vi "Make Timestamped Segment.vi"(0 "TreeNode in":refnum<class "TreeNode.lvclass">, 5 "Segment data":refnum<class "Data.lvclass">, 7 "Timestamps":refnum<class "Int64Array.lvclass">, 9 "Array":i64[](array[numeric]), 11 "error in (no error)":errorcluster) -> (4 "TreeNode out":refnum<class "TreeNode.lvclass">, 15 "error out":errorcluster)   [LabVIEW 2015, in "MDSplus.lvlib" / "TreeNode.lvclass"]
doc: "Write a single row of timestamped data."
uses:
  <vilib>/MDSplus/Classes/Data_Class/TreeNode_Class/TreeNode.lvclass
  <vilib>/MDSplus/Classes/Data_Class/Data.lvclass
  <vilib>/MDSplus/Classes/Data_Class/Array_Class/Int64Array_Class/Int64Array.lvclass
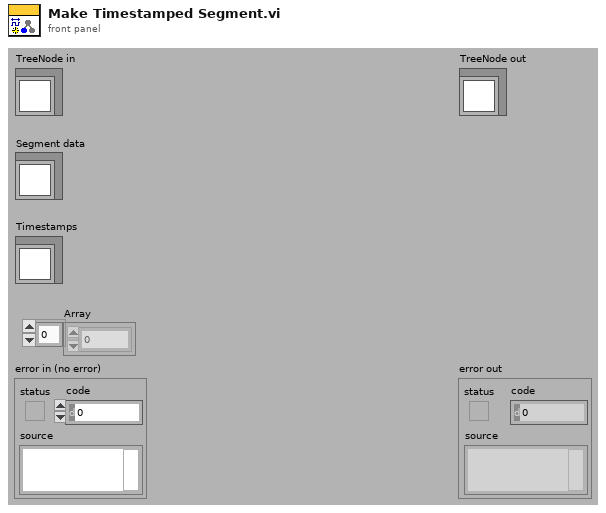
[diagram p1: front panel]
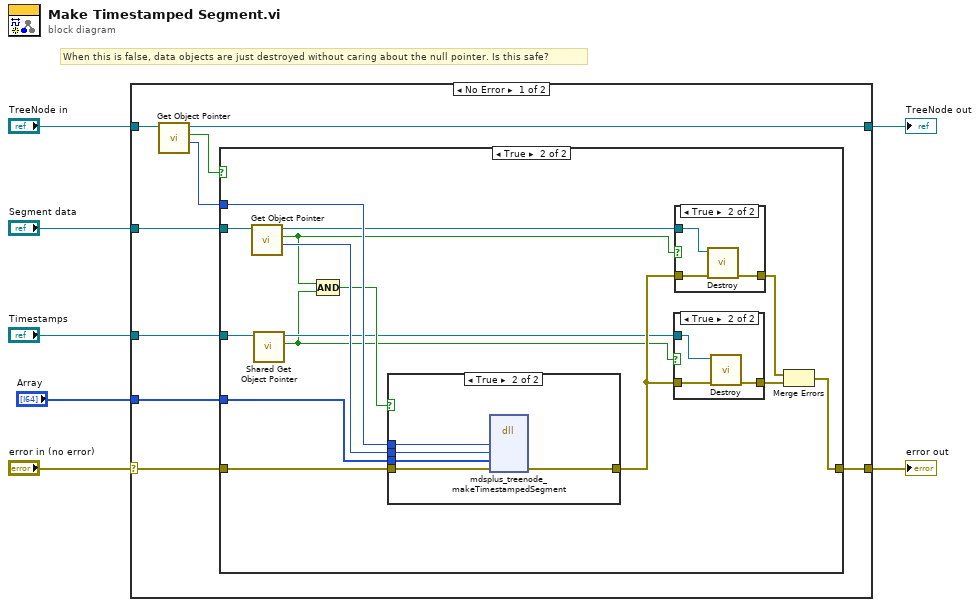
[diagram p0: block diagram]
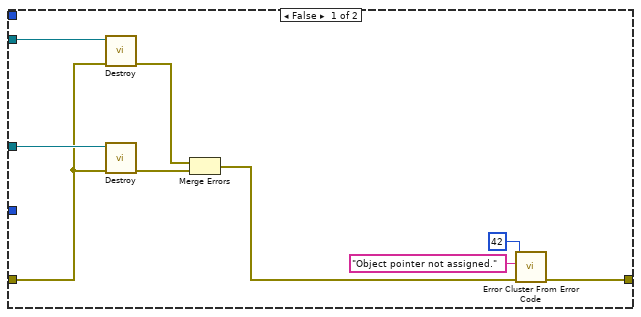
[diagram p2: hidden frame]
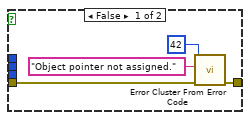
[diagram p5: hidden frame]
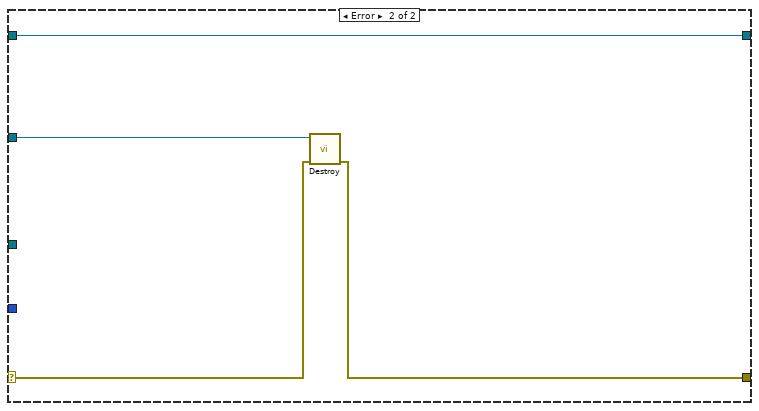
[diagram p6: hidden frame]
diagram:
  # "When this is false, data objects are just destroyed without caring about the null pointer. Is this safe?"
  n1 = case shown="No Error" "error in (no error)" {
    selector: "error in (no error)" -> [w12 w59]
    tunnel: [w11 w58] -> w6
    tunnel: [w10 w61] -> w4
    tunnel: "TreeNode in" -> [w16 w61]
    tunnel: "Segment data" -> [w15 w60]
    tunnel: "Timestamps" -> [w9 _]
    tunnel: "Array" -> [w8 _]
    frame No Error {
      n2 = call-dynamic "Get Object Pointer.vi"("Data in"=w16) -> ("Object Pointer"=w13:i64, "Assigned object pointer?"=w14:bool, "Data out"=w10:refnum<class "TreeNode.lvclass">)  [unwired: 8 in]
      n3 = case shown="True" w14 {
        tunnel: w15 -> [w22 w40]
        tunnel: w13 -> [_ w38]
        tunnel: w12 -> [w20 w37]
        tunnel: [w23 w27] -> w11
        tunnel: w9 -> [w21 w36]
        tunnel: w8 -> [_ w26]
        frame False {
          n4 = call-dynamic "Destroy.vi"("error in (no error)"=w20, "Data in"=w22) -> ("error out"=w19:errorcluster)  [unwired: 9 in]
          n5 = call-dynamic "Destroy.vi"("error in (no error)"=w20, "Int64Array in"=w21) -> ("error out"=w18:errorcluster)  [unwired: 9 in]
          n6 = Merge Errors(w19, w18) -> (w17:errorcluster)
          n7 = call <vilib>:"Error Cluster From Error Code.vi"("error in (no error)"=w17, "error message (\"\")"="Object pointer not assigned." ("error message (\"\")"), "error code (0)"=42) -> ("error out"=w23:errorcluster)  [unwired: 6 in]
        }
        frame True {
          n8 = call-dynamic "Get Object Pointer.vi"("Data in"=w40) -> ("Object Pointer"=w39:i64, "Assigned object pointer?"=w31:bool, "Data out"=w33:refnum<class "Data.lvclass">)  [unwired: 8 in]
          n9 = call <vilib>:"Shared Get Object Pointer.vi"("Data in"=w36) -> ("Assigned object pointer?"=w30:bool, "Data out"=w32:refnum<class "Int64Array.lvclass">)  [unwired: 8 in, 1 out]
          n10 = Compound Arithmetic op=AND(w31, w30) -> (w35:bool)
          n11 = case shown="True" w35 {
            tunnel: w39 -> [_ w53]
            tunnel: w38 -> [_ w56]
            tunnel: w37 -> [w49 w57]
            tunnel: [w50 w54] -> w34
            tunnel: w26 -> [_ w55]
            frame False {
              n12 = call <vilib>:"Error Cluster From Error Code.vi"("error in (no error)"=w49, "error message (\"\")"="Object pointer not assigned." ("error message (\"\")"), "error code (0)"=42) -> ("error out"=w50:errorcluster)  [unwired: 6 in]
            }
            frame True {
              n13 = dll-call lib="MDSobjectsLVShr" fn="mdsplus_treenode_makeTimestampedSegment"("lvTreeNodePtr"=w56, "lvArrayPtrIn"=w53, "lvLngArrHdlIn"=w55, "error"=w57) -> ("error"=w54:errorcluster)  [unwired: 7 in, 2 out]
            }
          }
          n14 = case shown="True" w30 {
            tunnel: w34 -> [w45 w48]
            tunnel: w32 -> [_ w46]
            tunnel: [w45 w47] -> w28
            frame False {
            }
            frame True {
              n15 = call-dynamic "Destroy.vi"("error in (no error)"=w48, "Int64Array in"=w46) -> ("error out"=w47:errorcluster)  [unwired: 9 in]
            }
          }
          n16 = case shown="True" w31 {
            tunnel: w34 -> [w41 w44]
            tunnel: w33 -> [_ w43]
            tunnel: [w41 w42] -> w29
            frame False {
            }
            frame True {
              n17 = call-dynamic "Destroy.vi"("error in (no error)"=w44, "Data in"=w43) -> ("error out"=w42:errorcluster)  [unwired: 9 in]
            }
          }
          n18 = Merge Errors(w29, w28) -> (w27:errorcluster)
        }
      }
    }
    frame Error {
      n19 = call-dynamic "Destroy.vi"("error in (no error)"=w59, "Data in"=w60) -> ("error out"=w58:errorcluster)  [unwired: 9 in]
    }
  }
  "error out" <- w6
  "TreeNode out" <- w4
